vi "Destroy Q.vi"(8 "error in (no error)":errorcluster) -> (0 "error out":errorcluster)   [LabVIEW 2017, in "Messaging Library.lvlib"]
uses:
  Messaging Library.lvlib
  Controls/Q FGV States.ctl
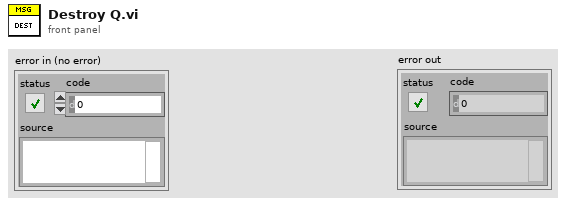
[diagram p1: front panel]
types:
  T1 = typedef "Messaging Library.lvlib/Q FGV States.ctl" = enum16{"Set", "Get"}
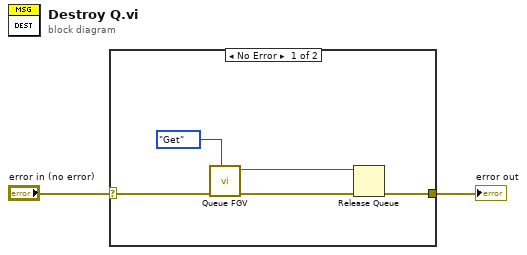
[diagram p0: block diagram]
diagram:
  n1 = case shown="No Error" "error in (no error)" {
    selector: "error in (no error)" -> [w6 w8]
    tunnel: [w7 w8] -> w1
    frame No Error {
      n2 = call "Queue FGV.vi"("States"=Q_FGV_States."Get", "error in (no error)"=w6) -> ("error out"=w5:errorcluster, "Message Q Out"=w4:refnum<queue>)  [unwired: 8 in]
      n3 = Release Queue(queue=w4, error in (no error)=w5) -> (error out=w7:errorcluster)  [unwired: 1 in, 2 out]
    }
    frame Error {
    }
  }
  "error out" <- w1
